vi "top_level.vi"() -> ()   [LabVIEW 2010]
panel:
  in  "Write to terminal":bool
  out "Boolean":bool
  # "This vi executes incorrectly if the sub vi pannel is open \nand you are only writing to the local variable in the sub VI"
  # "This boolean should always be true"
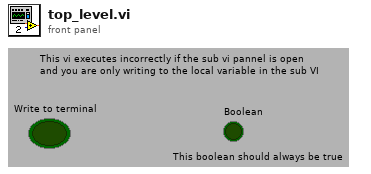
[diagram p1: front panel]
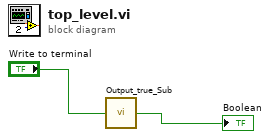
[diagram p0: block diagram]
diagram:
  n1 = call "Output_true_Sub.vi"("Write to terminal"="Write to terminal") -> ("Boolean"=→"Boolean":bool)
